vi "FTW-Endpoint-Multipart-Ask.vi"(0 "FTW Endpoint":refnum<class "FTW-Endpoint.lvclass">, 5 "Multipart Message":string[](array[string]), 7 "Read Timeout":i32=100 format="%dmsec", 9 "Write Timeout":i32 format="%dmsec", 11 "error in":errorcluster) -> (4 "FTW Endpoint out":refnum<class "FTW-Endpoint.lvclass">, 6 "Reply":string[](array[string]), 8 "Read Timed out?":bool, 10 "Write Timed out?":bool, 15 "error out":errorcluster)   [LabVIEW 2012, in "FTW-Actor.lvlib" / "FTW-Endpoint.lvclass"]
uses:
  FTW-Endpoint.lvclass
  FTW-Endpoint.lvclass/FTW-Endpoint.ctl
  Ether/FTW-Ether.lvclass
panel:
  # "Inputs"
  # "Outputs"
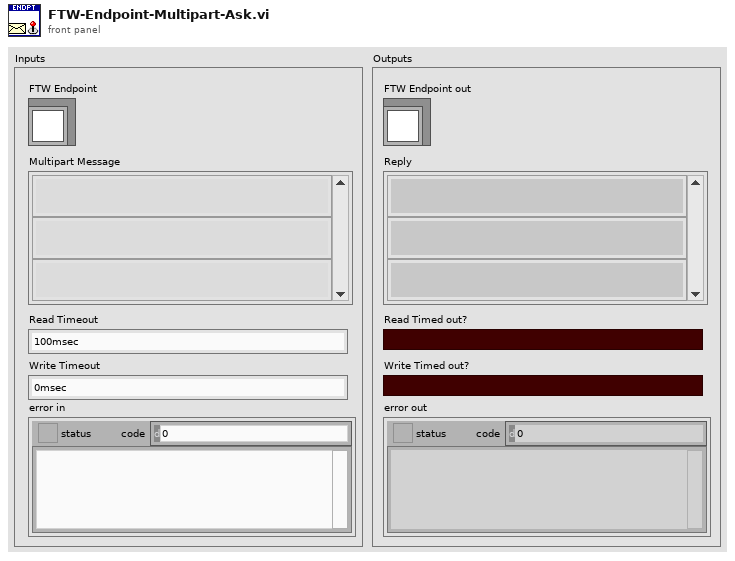
[diagram p1: front panel]
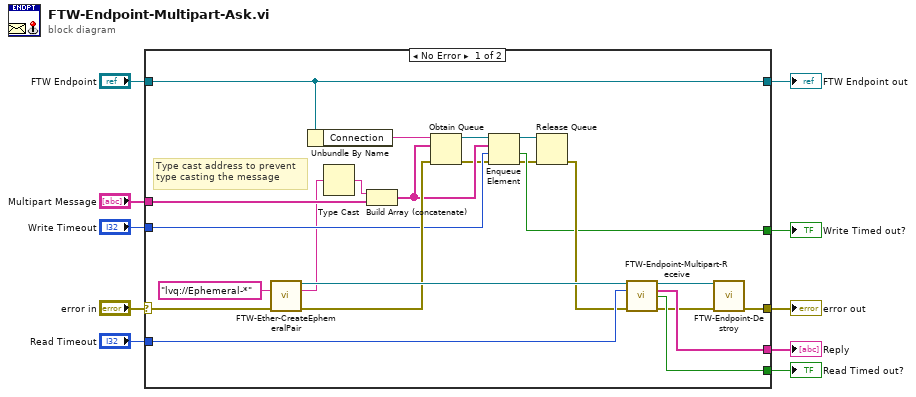
[diagram p0: block diagram]
diagram:
  n1 = case shown="No Error" "error in" {
    selector: "error in" -> [w32 w35]
    tunnel: [w25 w35] -> w10
    tunnel: [w20 w34] -> w8
    tunnel: "FTW Endpoint" -> [w20 w34]
    tunnel: "Multipart Message" -> [w33 _]
    tunnel: "Read Timeout" -> [w30 _]
    tunnel: [w28 _] -> w4
    tunnel: [w29 _] -> w3
    tunnel: [w21 _] -> w2
    tunnel: "Write Timeout" -> [w19 _]
    frame No Error {
      # "Type cast address to prevent\ntype casting the message"
      n2 = call "FTW-Ether-CreateEphemeralPair.vi"("Requested Ephemeral Address"="lvq://Ephemeral-*", "error in"=w32) -> ("Ephemeral Endpoint"=w31:refnum<class "FTW-Endpoint.lvclass">, "Actual Ephemeral Address"=w12:string, "error out"=w23:errorcluster)  [unwired: 11 in]
      n3 = Unbundle By Name(w20) -> ("Connection"=w15:string)
      n4 = Type Cast(x=w12) -> (*(type *) &x=w11:string)  [unwired: 1 in]
      n5 = Build Array (concatenate)(w11, w33) -> (w18:string[])
      n6 = Obtain Queue(name (unnamed)=w15, element data type=w18, error in (no error)=w23) -> (queue out=w16:refnum<queue>, error out=w17:errorcluster)  [unwired: 2 in, 1 out]
      n7 = Enqueue Element(queue=w16, element=w18, timeout in ms (-1)=w19, error in (no error)=w17) -> (queue out=w14:refnum<queue>, timed out?=w21:bool, error out=w13:errorcluster)
      n8 = Release Queue(queue=w14, error in (no error)=w13) -> (error out=w22:errorcluster)  [unwired: 1 in, 2 out]
      n9 = call-dynamic "FTW-Endpoint-Multipart-Receive.vi"("FTW Endpoint"=w31, "Timeout"=w30, "error in"=w22) -> ("FTW Endpoint out"=w27:refnum<class "FTW-Endpoint.lvclass">, "Message Received"=w29:string[], "Timed out?"=w28:bool, "error out"=w26:errorcluster)  [unwired: 9 in]
      n10 = call-dynamic "FTW-Endpoint-Destroy.vi"("FTW Endpoint"=w27, "error in"=w26) -> ("error out"=w25:errorcluster)  [unwired: 13 in]
    }
    frame Error {
    }
  }
  "error out" <- w10
  "FTW Endpoint out" <- w8
  "Read Timed out?" <- w4
  "Reply" <- w3
  "Write Timed out?" <- w2
